vi "Untitled 14.vi"() -> ()   [LabVIEW 2012]
uses:
  Global1.vi
  <vilib>/addons/database/Connection.llb/DB Tools Open Connec (Path).vi
  <vilib>/addons/_office/excel.llb/Excel Get Data (str).vi
  <vilib>/Utility/NIReport.llb/NI_report.lvclass
  <vilib>/Utility/NIReport.llb/Excel/NI_Excel.lvclass
  <vilib>/addons/_office/NI_ReportGenerationToolkit.lvlib
  <vilib>/addons/database/NI_Database_API.lvlib
panel:
  out "Numeric":i32
  in  "start (0, 0)":cluster{"start row":i32, "start column":i32}
  out "Numeric 2":i32
  in  "template (empty)":path=path "C:/m100/早車必回-1104.xls"
  out "row":i32
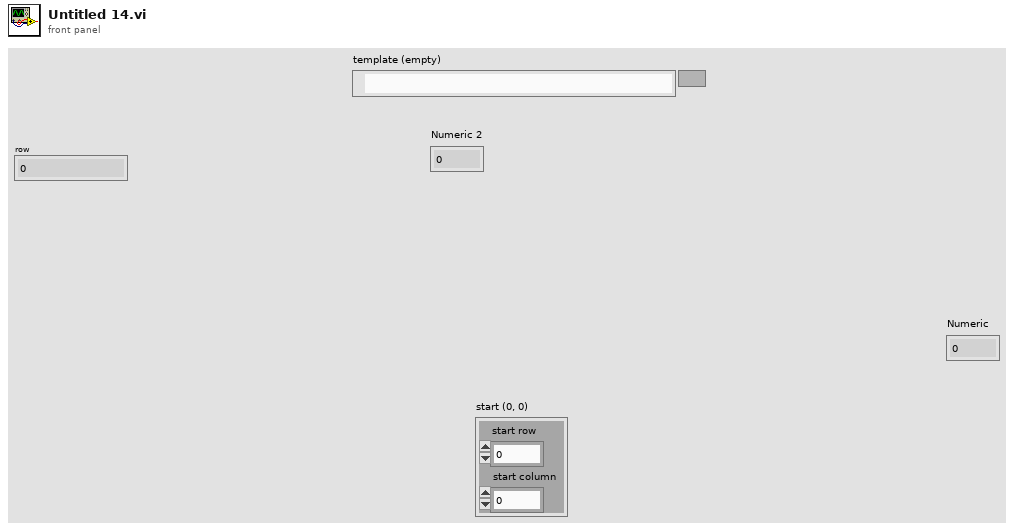
[diagram p1: front panel]
types:
  T1 = enum16{"Standard Report", "HTML", "Word", "Excel"}
  T2 = typedef "NI_Database_API.lvlib/Conn ObjectReference.ctl" = refnum<k1>
  T3 = cluster{"on/off":bool, "weight":i32, "color":u32}
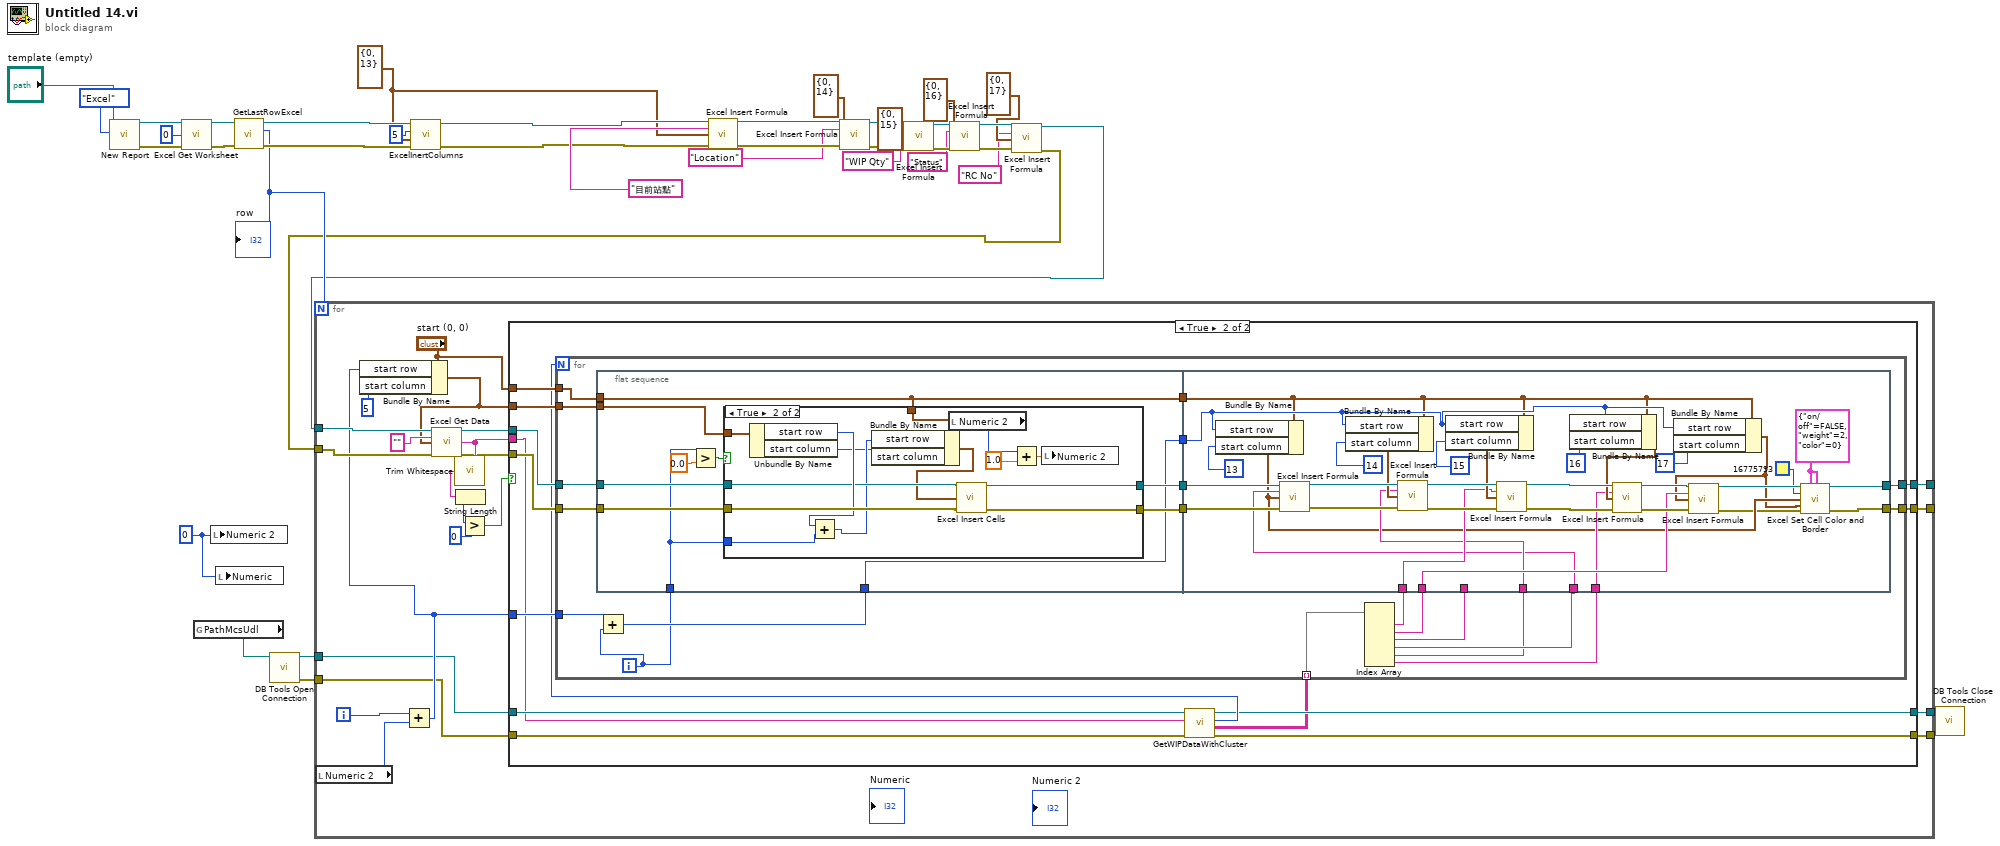
[diagram p0: block diagram]
diagram:
  w12 = 0
  w16 = cluster{"row":i32, "column":i32} {"row"=0, "column"=13} ("start (0, 0)")
  n1 = call <vilib>:"New Report.vi"("report type"=T1."Excel" ("Report Type"), "template (empty)"="template (empty)") -> ("report out"=w38:refnum<class "NI_report.lvclass">, "error out"=w37:errorcluster)  [unwired: 12 in]
  n2 = call <vilib>:"Excel Get Worksheet.vi"("report in"=w38, "worksheet index (0)"=0, "error in (no error)"=w37) -> ("report out"=w29:refnum<class "NI_report.lvclass">, "error out"=w28:errorcluster)  [unwired: 11 in]
  n3 = global read "Global1.vi" "PathMcsUdl"() -> (w7:path)
  n4 = local write "Numeric 2"(w12) -> ()
  n5 = local write "Numeric"(w12) -> ()
  n6 = call "GetLastRowExcel.vi"("error in (no error)"=w28, "report in"=w29) -> ("error out"=w20:errorcluster, "row"=w13:i32, "report out"=w21:refnum<class "NI_report.lvclass">)  [unwired: 7 in]
  "row" <- w13
  n7 = call-poly <vilib>:"DB Tools Open Connection.vi"("connection information"=w7) -> ("error out"=w10:errorcluster, "connection reference"=w11:T2)  [unwired: 7 in]
  n8 = call "ExcelInertColumns.vi"("error in (no error)"=w20, "start (0, 0)"=w16, "Numeric"=5, "report in"=w21) -> ("error out"=w17:errorcluster, "report out"=w18:refnum<class "NI_report.lvclass">)  [unwired: 6 in]
  n9 = call <vilib>:"Excel Insert Formula.vi"("report in"=w18, "formula"="目前站點", "start (0, 0)"=w16, "error in (no error)"=w17) -> ("report out"=w36:refnum<class "NI_report.lvclass">, "error out"=w34:errorcluster)  [unwired: 10 in]
  n10 = call <vilib>:"Excel Insert Formula.vi"("report in"=w36, "formula"="Location", "start (0, 0)"=cluster{"row":i32, "column":i32} {"row"=0, "column"=14}, "error in (no error)"=w34) -> ("report out"=w35:refnum<class "NI_report.lvclass">, "error out"=w33:errorcluster)  [unwired: 10 in]
  n11 = call <vilib>:"Excel Insert Formula.vi"("report in"=w35, "formula"="WIP Qty", "start (0, 0)"=cluster{"row":i32, "column":i32} {"row"=0, "column"=15}, "error in (no error)"=w33) -> ("report out"=w27:refnum<class "NI_report.lvclass">, "error out"=w26:errorcluster)  [unwired: 10 in]
  n12 = call <vilib>:"Excel Insert Formula.vi"("report in"=w27, "formula"="Status", "start (0, 0)"=cluster{"row":i32, "column":i32} {"row"=0, "column"=16}, "error in (no error)"=w26) -> ("report out"=w6:refnum<class "NI_report.lvclass">, "error out"=w5:errorcluster)  [unwired: 10 in]
  n13 = call <vilib>:"Excel Insert Formula.vi"("report in"=w6, "formula"="RC No", "start (0, 0)"=cluster{"row":i32, "column":i32} {"row"=0, "column"=17}, "error in (no error)"=w5) -> ("report out"=w1:refnum<class "NI_report.lvclass">, "error out"=w2:errorcluster)  [unwired: 10 in]
  n14 = for {
    N: w13 -> [_]
    tunnel: w1 -> [w59]
    tunnel: w2 -> [w58]
    tunnel: [w49] -> _
    tunnel: [w48] -> _
    tunnel: w11 -> [w43]
    tunnel: w10 -> [w42]
    tunnel: [w41] -> w9
    tunnel: [w40] -> w8
    i -> [w47]
    n15 = local read "Numeric 2"() -> (w46:i32)
    n16 = Add(x=w47, y=w46) -> (x+y=w45:i32)
    n17 = Bundle By Name(cluster="start (0, 0)", "start row"=w45, "start column"=5) -> (w44:cluster{"start row":i32, "start column":i32})
    n18 = call-poly <vilib>:"Excel Get Data.vi"("report in"=w59, "data type"="", "start (0, 0)"=w44, "error in (no error)"=w58) -> ("report out"=w51:refnum<class "NI_report.lvclass">, "data"=w53:string, "error out"=w50:errorcluster)  [unwired: 9 in]
    n19 = call <vilib>:"Trim Whitespace.vi"("string"=w53) -> ("trimmed string"=w56:string)  [unwired: 1 in]
    n20 = String Length(string=w56) -> (length=w55:i32)
    n21 = Greater?(x=w55, y=0) -> (0:w54:bool)
    n22 = case shown="True" w54 {
      tunnel: w53 -> [_ w70]
      tunnel: "start (0, 0)" -> [_ w79]
      tunnel: w51 -> [w65 w78]
      tunnel: w50 -> [w64 w77]
      tunnel: [w65 w76] -> w49
      tunnel: [w64 w75] -> w48
      tunnel: w45 -> [_ w74]
      tunnel: w44 -> [_ w73]
      tunnel: w43 -> [w63 w72]
      tunnel: w42 -> [w62 w71]
      tunnel: [w63 w68] -> w41
      tunnel: [w62 w67] -> w40
      frame False {
      }
      frame True {
        n23 = call "GetWIPDataWithCluster.vi"("error in"=w71, "Lotno"=w70, "connection reference"=w72) -> ("error out"=w67:errorcluster, "output array"=w66:string[][], "data"=w69:i32, "connection reference 2"=w68:T2)  [unwired: 5 in]
        n24 = for {
          N: w69 -> [_]
          tunnel: w78 -> [w99]
          tunnel: [w98] -> w76
          tunnel: w79 -> [w97]
          tunnel: w77 -> [w96]
          tunnel: [w95] -> w75
          tunnel: w74 -> [w94]
          tunnel: w73 -> [w88]
          tunnel: w66 -> [w87] mode=indexing
          i -> [w86]
          n25 = flat-sequence {
            tunnel: w99 -> [w104]
            tunnel: w97 -> [w101]
            tunnel: [w101] -> w92
            tunnel: w96 -> [w103]
            tunnel: w93 -> [w105]
            tunnel: [w105] -> w91
            tunnel: [w107] -> w90
            tunnel: [w106] -> w89
            tunnel: w86 -> [w100]
            tunnel: w88 -> [w102]
            tunnel: w92 -> [w139]
            tunnel: w91 -> [w142]
            tunnel: [w132] -> w98
            tunnel: w90 -> [w145]
            tunnel: [w131] -> w95
            tunnel: w89 -> [w144]
            tunnel: w85 -> [w138]
            tunnel: w84 -> [w137]
            tunnel: w83 -> [_]
            tunnel: w82 -> [w135]
            tunnel: w81 -> [w136]
            tunnel: w80 -> [w134]
            frame #0 {
              n26 = Greater?(x=w100, y=0.0) -> (0:w108:bool)
              n27 = case shown="True" w108 {
                tunnel: [w111 w125] -> w107
                tunnel: [w110 w124] -> w106
                tunnel: w104 -> [w111 w117]
                tunnel: w103 -> [w110 w120]
                tunnel: w102 -> [_ w119]
                tunnel: w101 -> [_ w116]
                tunnel: w100 -> [_ w112]
                frame False {
                }
                frame True {
                  n28 = Unbundle By Name(w119) -> ("start row"=w118:i32, "start column"=w114:i32)
                  n29 = Add(x=w118, y=w112) -> (x+y=w115:i32)
                  n30 = Bundle By Name(cluster=w116, "start row"=w115, "start column"=w114) -> (w113:cluster{"start row":i32, "start column":i32})
                  n31 = local read "Numeric 2"() -> (w123:i32)
                  n32 = call <vilib>:"Excel Insert Cells.vi"("report in"=w117, "start (0, 0)"=w113, "error in (no error)"=w120) -> ("report out"=w125:refnum<class "NI_report.lvclass">, "error out"=w124:errorcluster)  [unwired: 11 in]
                  n33 = Add(x=w123, y=1.0) -> (x+y=w121:dbl)
                  n34 = local write "Numeric 2"(w121) -> ()
                }
              }
            }
            frame #1 {
              w126 = T3 {"on/off"=FALSE, "weight"=2, "color"=0} ("inside border")
              n35 = Bundle By Name(cluster=w139, "start row"=w142, "start column"=13) -> (w129:cluster{"start row":i32, "start column":i32})
              n36 = call <vilib>:"Excel Insert Formula.vi"("report in"=w145, "formula"=w135, "start (0, 0)"=w129, "error in (no error)"=w144) -> ("report out"=w155:refnum<class "NI_report.lvclass">, "error out"=w152:errorcluster)  [unwired: 10 in]
              n37 = Bundle By Name(cluster=w139, "start row"=w142, "start column"=14) -> (w150:cluster{"start row":i32, "start column":i32})
              n38 = call <vilib>:"Excel Insert Formula.vi"("report in"=w155, "formula"=w136, "start (0, 0)"=w150, "error in (no error)"=w152) -> ("report out"=w154:refnum<class "NI_report.lvclass">, "error out"=w153:errorcluster)  [unwired: 10 in]
              n39 = Bundle By Name(cluster=w139, "start row"=w142, "start column"=15) -> (w151:cluster{"start row":i32, "start column":i32})
              n40 = call <vilib>:"Excel Insert Formula.vi"("report in"=w154, "formula"=w138, "start (0, 0)"=w151, "error in (no error)"=w153) -> ("report out"=w148:refnum<class "NI_report.lvclass">, "error out"=w147:errorcluster)  [unwired: 10 in]
              n41 = Bundle By Name(cluster=w139, "start row"=w142, "start column"=16) -> (w146:cluster{"start row":i32, "start column":i32})
              n42 = call <vilib>:"Excel Insert Formula.vi"("report in"=w148, "formula"=w134, "start (0, 0)"=w146, "error in (no error)"=w147) -> ("report out"=w141:refnum<class "NI_report.lvclass">, "error out"=w140:errorcluster)  [unwired: 10 in]
              n43 = Bundle By Name(cluster=w139, "start row"=w142, "start column"=17) -> (w127:cluster{"start row":i32, "start column":i32})
              n44 = call <vilib>:"Excel Insert Formula.vi"("report in"=w141, "formula"=w137, "start (0, 0)"=w127, "error in (no error)"=w140) -> ("report out"=w133:refnum<class "NI_report.lvclass">, "error out"=w128:errorcluster)  [unwired: 10 in]
              n45 = call <vilib>:"Excel Set Cell Color and Border.vi"("report in"=w133, "inside border"=w126, "outside border"=w126, "background color (w)"=u32 16775793, "start (-1, -1)"=w129, "end (-1, -1)"=w127, "error in (no error)"=w128) -> ("report out"=w132:refnum<class "NI_report.lvclass">, "error out"=w131:errorcluster)  [unwired: 7 in]
            }
          }
          n46 = Add(x=w94, y=w86) -> (x+y=w93:i32)
          n47 = Index Array(array=w87) -> (element #1=w85:string, element #2=w84:string, element #3=w83:string, element #4=w82:string, element #5=w81:string, element #6=w80:string)  [unwired: 6 in]
        }
      }
    }
  }
  n48 = call <vilib>:"DB Tools Close Connection.vi"("error in (no error)"=w8, "connection reference"=w9) -> ()  [unwired: 5 in, 1 out]
